vi "Write LogFile Path.vi"(8 "error in":errorcluster, 10 "LogFile Directory":path, 11 "Console Log in":refnum<class "Console Log.lvclass">) -> (0 "error out":errorcluster, 3 "Console Log out":refnum<class "Console Log.lvclass">)   [LabVIEW 2011, in "Console Log.lvclass"]
uses:
  Console Log.lvclass
  Console Log.lvclass/Console Log.ctl
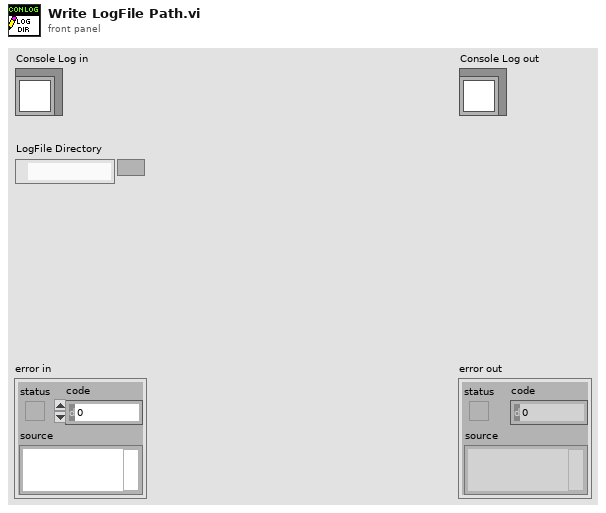
[diagram p1: front panel]
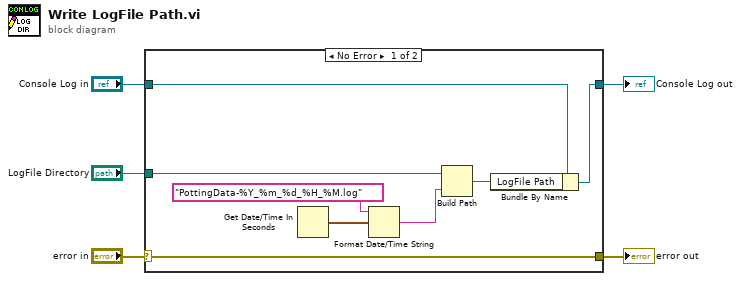
[diagram p0: block diagram]
diagram:
  n1 = case shown="No Error" "error in" {
    selector: "error in" -> [w13 w14]
    tunnel: [w13 w14] -> w4
    tunnel: [w11 w15] -> w2
    tunnel: "Console Log in" -> [w12 w15]
    tunnel: "LogFile Directory" -> [w8 _]
    frame No Error {
      n2 = Get Date/Time In Seconds() -> (seconds since 1Jan1904=w10:timestamp)
      n3 = Format Date/Time String(time format string (%c)="PottingData-%Y_%m_%d_%H_%M.log", seconds (now)=w10) -> (date/time string=w6:string)  [unwired: 1 in]
      n4 = Build Path(base path=w8, name or relative path=w6) -> (appended path=w7:path)
      n5 = Bundle By Name(cluster=w12, "LogFile Path"=w7) -> (w11:refnum<class "Console Log.lvclass">)
    }
    frame Error {
    }
  }
  "error out" <- w4
  "Console Log out" <- w2
